vi "unflattenAccelerationFromXML_Scalar.vi"(8 "error in (no error)":errorcluster, 9 "accelerationUnitInXML":T1, 10 "xmlString":string, 11 "accelerationForType":dbl[unit]) -> (0 "error out":errorcluster, 3 "acceleration":dbl[unit])   [LabVIEW 2016, in "UnitsAndXML.lvlib"]
uses:
  <userlib>/Common/UnitsAndXML/UnitsAndXML.lvlib
  <userlib>/Common/UnitsAndXML/FlattenItemWithUnitToXML/FlattenAccelerationToXML/AccelerationUnit.ctl
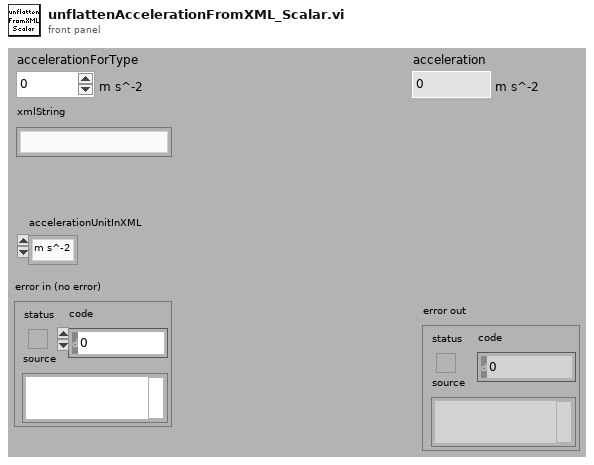
[diagram p1: front panel]
types:
  T1 = typedef "UnitsAndXML.lvlib/AccelerationUnit.ctl" = enum16{"m s^-2"}
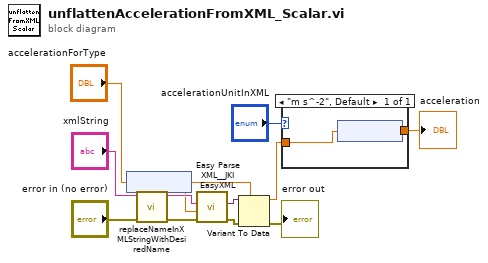
[diagram p0: block diagram]
diagram:
  n1 = node("accelerationForType") -> (w7:dbl)
  n2 = call <userlib>:"replaceNameInXMLStringWithDesiredName.vi"("error in"="error in (no error)", "xmlString"="xmlString") -> ("error out"=w1:errorcluster, "revisedXMLString"=w9:string)  [unwired: 8 in]
  n3 = call <vilib>:"Easy Parse XML__JKI EasyXML.vi"("error in (no error)"=w1, "LabVIEW Data (Type)"=w7, "XML String"=w9) -> ("error out"=w4:errorcluster, "LabVIEW Data"=w11:variant)  [unwired: 7 in]
  n4 = Variant To Data(error in=w4, type=w7, Variant=w11) -> (data=w6:dbl, error out=→"error out":errorcluster)
  n5 = case shown="\"m s^-2\", Default" "accelerationUnitInXML" {
    tunnel: w6 -> [w14]
    tunnel: [w13] -> w5
    frame "m s^-2", Default {
      n6 = node(w14) -> (w13:dbl[unit])
    }
  }
  "acceleration" <- w5
